vi "파일IO.vi"() -> ()   [LabVIEW 2014]
uses:
  <vilib>/Utility/file.llb/Write To Spreadsheet File (DBL).vi
  <vilib>/Analysis/NI_AALBase.lvlib
panel:
  out "웨이브폼 그래프":dbl[][](graph)
  in  "파일 경로(대화 상자 사용)":path
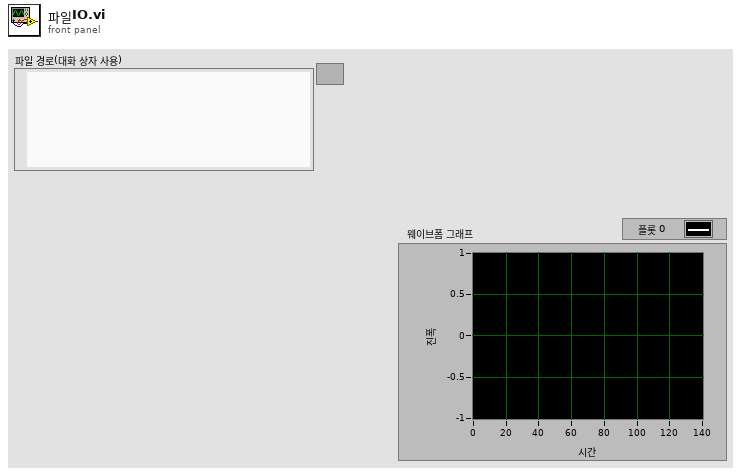
[diagram p1: front panel]
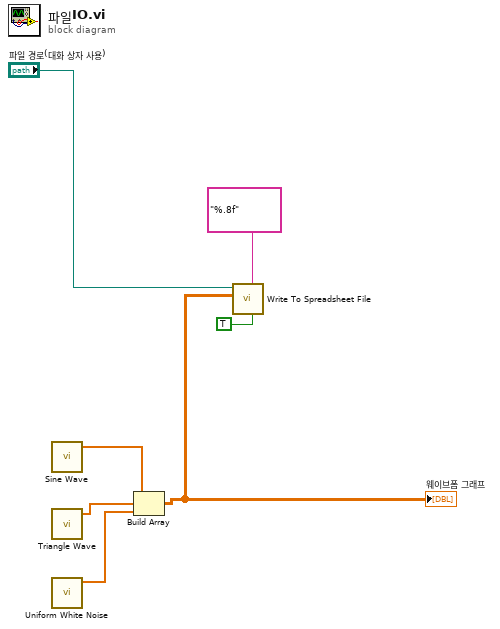
[diagram p0: block diagram]
diagram:
  n1 = call <vilib>:"Sine Wave.vi"() -> ("sine wave"=w7:dbl[])  [unwired: 5 in, 2 out]
  n2 = call <vilib>:"Triangle Wave.vi"() -> ("triangle wave"=w6:dbl[])  [unwired: 5 in, 2 out]
  n3 = call <vilib>:"Uniform White Noise.vi"() -> ("uniform white noise"=w5:dbl[])  [unwired: 10 in, 1 out]
  n4 = Build Array(w7, w6, w5) -> (w4:dbl[][])
  "웨이브폼 그래프" <- w4
  n5 = call-poly <vilib>:"Write To Spreadsheet File.vi"("transpose? (no:F)"=TRUE, "format (%.3f)"="%.8f", "2D data"=w4, "file path (dialog if empty)"="파일 경로(대화 상자 사용)") -> ()  [unwired: 4 in, 1 out]
